vi "CreateTasks.vi"(8 "error in (no error)":errorcluster, 11 "DAQ_Module in":refnum<class "DAQ_Module.lvclass">) -> (0 "error out":errorcluster, 3 "DAQ_Module out":refnum<class "DAQ_Module.lvclass">)   [LabVIEW 2025, in "DAQ_Module.lvlib" / "DAQ_Module.lvclass"]
uses:
  DAQ_Module.lvclass
  <vilib>/ActorFramework/Message Enqueuer/Message Enqueuer.lvclass
  DAQ_Module Messages/RefreshList Msg/RefreshList Msg.lvclass
  <vilib>/ActorFramework/Actor/Actor.lvclass/Actor.ctl
  <vilib>/ActorFramework/Message Enqueuer/Message Enqueuer.lvclass/Message Enqueuer.ctl
  DAQ_Module.lvclass/DAQ_Module.ctl
  Read TaskConfig.vi
  <vilib>/ActorFramework/Message Enqueuer/Init from Existing Queue.vi
  <vilib>/ActorFramework/Actor/Actor.lvclass
  <vilib>/ActorFramework/Actor Framework.lvlib
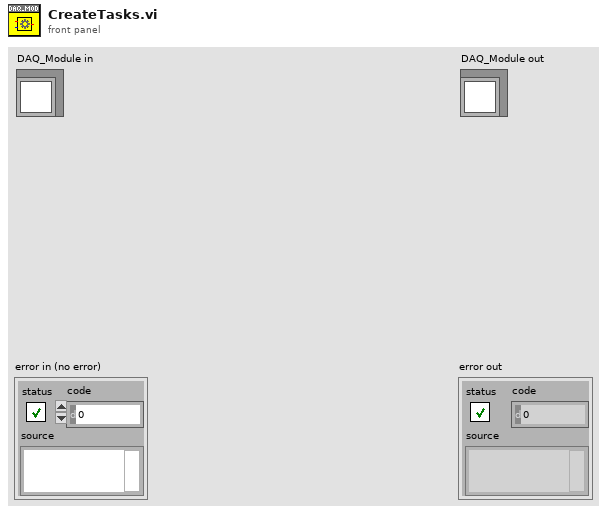
[diagram p1: front panel]
types:
  T1 = map{string, refnum<class "Message Enqueuer.lvclass">}
  T2 = typedef "DAQ_Module.lvlib/DAQ_Module.lvclass/DAQ_Config.ctl" = map{string, T3}
  T3 = typedef "DAQ_Module.lvlib/DAQ_Module.lvclass/DAQ_Task_Config.ctl" = cluster{"Drive":T4, "TaskType":T5, "PhysicalChannels":string, "SampleRateConfiguration":T6, "ChannelConfig":string, "Enable":bool, "ShowPanel":bool}
  T4 = typedef "DAQ_Module.lvlib/DAQ_Module.lvclass/DAQ_HW_Type.ctl" = enum16{"NI_DAQmx", "Simulated_DAQ"}
  T5 = typedef "DAQ_Module.lvlib/DAQ_Module.lvclass/DAQ_Task_Type.ctl" = enum16{"AI", "Linear", "Angular", "AO"}
  T6 = typedef "DAQ_Module.lvlib/DAQ_Module.lvclass/DAQ_SampleRateConfig.ctl" = cluster{"SampleRate":dbl, "SamplesPerChannel":u32, "SamplesPerRead":i32, "SampleMode":i32, "Clock Source":string}
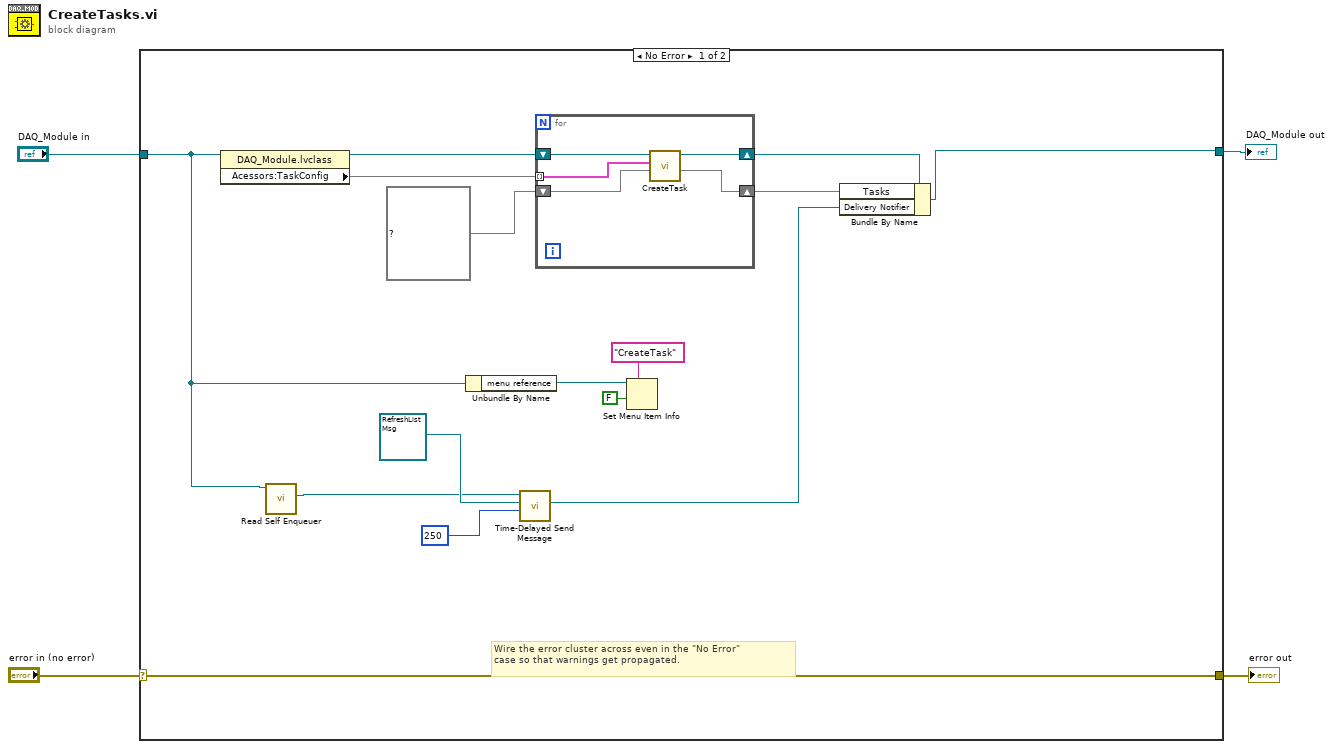
[diagram p0: block diagram]
diagram:
  n1 = case shown="No Error" "error in (no error)" {
    selector: "error in (no error)" -> [w19 w26]
    tunnel: [w19 w26] -> w3
    tunnel: [w10 w25] -> w1
    tunnel: "DAQ_Module in" -> [w9 w25]
    frame No Error {
      # "Wire the error cluster across even in the \"No Error\"\ncase so that warnings get propagated."
      n2 = property class="DAQ_Module.lvclass"(reference=w9) -> (reference out=w17:refnum<class "DAQ_Module.lvclass">, "Acessors:TaskConfig"=w18:T2)  [unwired: 1 in, 1 out]
      n3 = call <vilib>:"Read Self Enqueuer.vi"("Actor"=w9) -> ("Self Enqueuer"=w6:refnum<class "Message Enqueuer.lvclass">)  [unwired: 10 in]
      n4 = Unbundle By Name(w9) -> ("menu reference"=w13:refnum<k9>)
      n5 = call <vilib>:"Time-Delayed Send Message.vi"("Milliseconds To Wait"=250, "Message"=refnum<class "RefreshList Msg.lvclass"> refnum ("DAQ_Module.lvlib:RefreshList Msg.lvclass"), "Message Enqueuer"=w6) -> ("Delivery Notifier"=w5:refnum<notifier>)  [unwired: 7 in, 1 out]
      n6 = for {
        tunnel: w18 -> [w23] mode=indexing
        shift-right: [w21] -> w15
        shift-left: w17 -> [w24]
        shift-right: [w20] -> w14
        shift-left: T1 {} ("Tasks") -> [w22]
        n7 = call "CreateTask.vi"("Tasks in"=w22, "Cluster"=w23, "DAQ_Module in"=w24) -> ("Tasks out"=w20:T1, "DAQ_Module out"=w21:refnum<class "DAQ_Module.lvclass">)  [unwired: 6 in, 1 out]
      }
      n8 = Set Menu Item Info(7:"CreateTask" ("item tag"), 9:FALSE ("enabled"), 11:w13) -> ()  [unwired: 4 in, 2 out]
      n9 = Bundle By Name(cluster=w15, "Tasks"=w14, "Delivery Notifier"=w5) -> (w10:refnum<class "DAQ_Module.lvclass">)
    }
    frame Error {
    }
  }
  "error out" <- w3
  "DAQ_Module out" <- w1
